vi "home.vi"() -> ()   [LabVIEW 2016]
uses:
  <vilib>/Platform/TimedLoop/XDataNode/timing_clust.ctl
  <vilib>/Platform/TimedLoop/XDataNode/nitl_modes.ctl
  <vilib>/Platform/TimedLoop/XDataNode/wakeup.ctl
  C:/Program Files (x86)/Real Games/Home IO/Home IO_Data/Plugins/EngineIO.dll
  <vilib>/platform/TimedLoop/XDataNode/XDataNode.xnode
  <vilib>/Platform/TimedLoop/XDataNode/XDNodeRunTimeDep.lvlib
panel:
  in  "Gain integrateur":dbl=3.0
  in  "Mode":bool
  in  "consigne luminosité":dbl(knob) scale=0.0..10.0
  out "error out":errorcluster
  out "Waveform Chart":T1(graph)
  in  "stop":bool
  in  "éclairage manuel":dbl(knob) scale=0.0..10.0
  in  "Te(ms)":i64=200
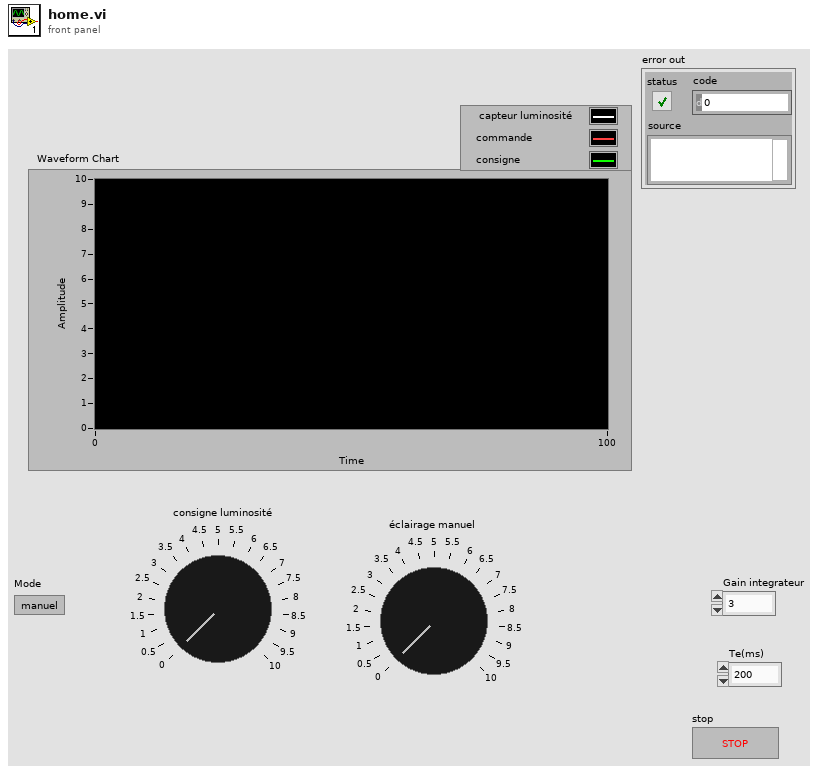
[diagram p1: front panel]
types:
  T1 = cluster{"Value":sgl, "upper limit":dbl, "consigne luminosité":dbl}
  T2 = typedef "XDNodeRunTimeDep.lvlib/timing_clust.ctl" = cluster{"Expected End [f-1]":u64, "Actual End [f-1]":u64, "Finished Late? [f-1]":bool, "Expected End [i-1]":u64, "Actual End [i-1]":u64, "Finished Late? [i-1]":bool, "Expected Start [i]":u64, "Actual Start [i]":u64, "Expected Start [f]":u64, "Actual Start [f]":u64, "Source Name":string, "Structure Name":string, "Period":i64, "Deadline":i64, "Offset":i64, "Start":i64, "Priority":i32, "Timeout":i32, "Mode":T3, "Wakeup Reason":T4, "Error":errorcluster, "Source Type":string, "Secondary Source Type":string, "Global End Time":u64, "Global Start Time":u64, "Frame Duration":u64, "Iteration Duration":u64, "Assigned CPU":i32, "I/O Scan Engine Mode":u32}
  T3 = typedef "XDNodeRunTimeDep.lvlib/nitl_modes.ctl" = enum32{"No Change", "Process missed periods, maintain original phase", "Discard missed periods, maintain original phase", "Process missed periods, ignore original phase", "Discard missed periods, ignore original phase"}
  T4 = typedef "XDNodeRunTimeDep.lvlib/wakeup.ctl" = enum32{"Normal", "Aborted", "Asynchronous wakeup", "Timing source error", "Timed loop error", "Timeout"}
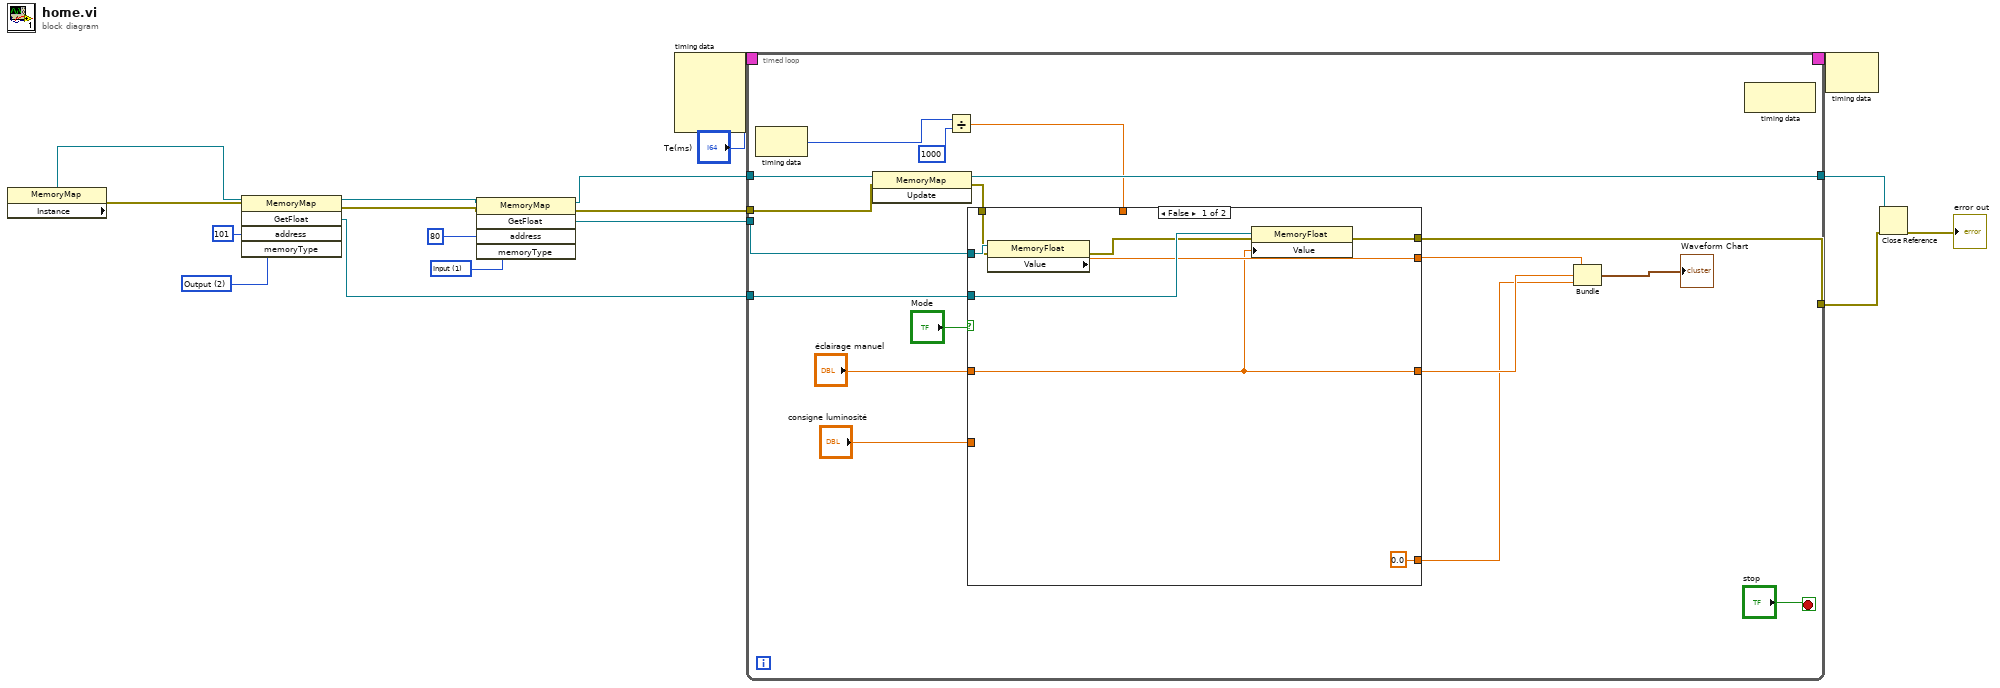
[diagram p0: block diagram]
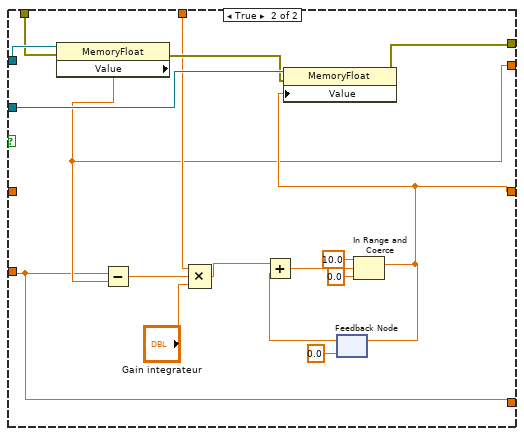
[diagram p2: hidden frame]
diagram:
  w14 = 1 items=["Memory", "Input", "Output"] ("memoryType")
  w16 = 2 items=["Memory", "Input", "Output"] ("memoryType")
  n1 = property class="MemoryMap"() -> (error out=w5:errorcluster, "Instance"=w18:refnum<k24>)  [unwired: 2 in, 1 out]
  n2 = invoke class="MemoryMap" method="GetFloat"(reference=w18, error in=w5, "address"=101, "memoryType"=w16) -> (reference out=w9:refnum<k24>, error out=w4:errorcluster, "GetFloat"=w7:refnum<k24>)  [unwired: 1 in, 2 out]
  n3 = invoke class="MemoryMap" method="GetFloat"(reference=w9, error in=w4, "address"=80, "memoryType"=w14) -> (reference out=w10:refnum<k24>, error out=w3:errorcluster, "GetFloat"=w8:refnum<k24>)  [unwired: 1 in, 2 out]
  n4 = node-c288("Te(ms)") -> (w13:T2)  [unwired: 3 in]
  n5 = timed-loop {
    timing: w13 -> [_]
    timing-out: [_] -> w12
    tunnel: w10 -> [w36]
    tunnel: w8 -> [w35]
    tunnel: w7 -> [w34]
    tunnel: [w30] -> w6
    tunnel: w3 -> [w29]
    tunnel: [w27] -> w2
    stop <- "stop" stop-if-true
    n6 = node-c288() -> (w22:i64)  [unwired: 1 in]
    n7 = invoke class="MemoryMap" method="Update"(reference=w36, error in=w29) -> (reference out=w30:refnum<k24>, error out=w28:errorcluster)  [unwired: 1 in, 1 out]
    n8 = Divide(x=w22, y=i64 1000) -> (x/y=w20:dbl)
    n9 = case shown="False" "Mode" {
      tunnel: w35 -> [w44 w61]
      tunnel: w34 -> [w43 w59]
      tunnel: [w42 w46] -> w32
      tunnel: w28 -> [w41 w60]
      tunnel: [w39 w57] -> w27
      tunnel: [w38 w47] -> w25
      tunnel: "éclairage manuel" -> [w38 _]
      tunnel: "consigne luminosité" -> [_ w45]
      tunnel: w20 -> [_ w54]
      tunnel: [0.0 ("consigne luminosité") w45] -> w19
      frame False {
        n10 = property class="MemoryFloat"(reference=w44, error in=w41) -> (error out=w40:errorcluster, "Value"=w42:sgl)  [unwired: 1 out]
        n11 = property class="MemoryFloat"(reference=w43, error in=w40, "Value"=w38) -> (error out=w39:errorcluster)  [unwired: 1 out]
      }
      frame True {
        n12 = property class="MemoryFloat"(reference=w61, error in=w60) -> (error out=w58:errorcluster, "Value"=w46:sgl)  [unwired: 1 out]
        n13 = Subtract(x=w45, y=w46) -> (x-y=w56:dbl)
        n14 = Compound Arithmetic op=MULTIPLY(w54, w56, "Gain integrateur") -> (w53:dbl)
        n15 = feedback #1(0.0 ("upper limit")) -> (w49:dbl)
        n16 = Add(x=w53, y=w49) -> (x+y=w52:dbl)
        n17 = In Range and Coerce(upper limit=10.0, x=w52, lower limit=0.0) -> (coerced(x)=w47:dbl)  [unwired: 1 out]
        n18 = property class="MemoryFloat"(reference=w59, error in=w58, "Value"=w47) -> (error out=w57:errorcluster)  [unwired: 1 out]
        n19 = feedback-in #1(w47) -> ()
      }
    }
    n20 = Bundle("Value"=w32, "upper limit"=w25, "consigne luminosité"=w19) -> (→"Waveform Chart":T1)  [unwired: 1 in]
    n21 = node-c288() -> ()  [unwired: 1 in, 1 out]
  }
  n22 = node-c288(w12) -> ()  [unwired: 1 out]
  n23 = Close Reference(reference=w6, error in (no error)=w2) -> (error out=→"error out":errorcluster)
